vi "e.gate HighSpeedPort Decode TimeStamp.vi"(0 "Data in (binary)":u8[](array[numeric]), 1 "Time Format String":string, 2 "dActTimeDataType":i32, 3 "StartTimeToDayFactor":dbl, 4 "dActTimeToSecondFactor":dbl, 5 "StartTime":dbl, 7 "error in (no error)":errorcluster, 15 "Array":dbl[](array[numeric])) -> (20 "OLE time":dbl, 21 "date time array (double)":dbl[](array[numeric]), 22 "date time cluster":T1 caption="date time rec", 27 "error out":cluster{"status":bool, i32, "source":string})   [LabVIEW 2016]
doc: "This VI is used to decode the timestamp of a buffer frame depending on calculated time information's from the controller and a Time Format String which defines the time/date information's to be inserted in the output array."
uses:
  <vilib>/Utility/miscctls.llb/LVDateTimeRec.ctl
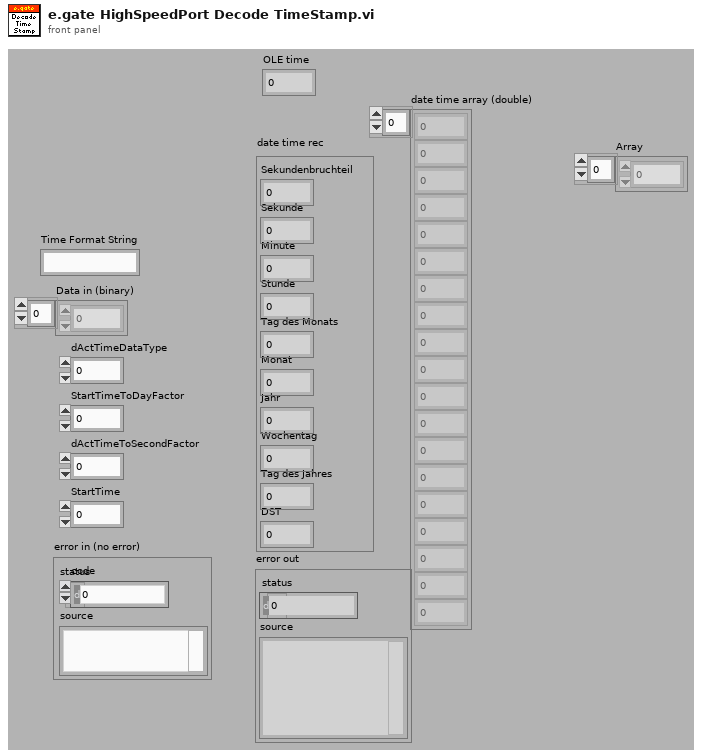
[diagram p1: front panel]
types:
  T1 = typedef "LVDateTimeRec.ctl" = cluster{"fractional second":dbl, "second":i32, "minute":i32, "hour":i32, "day of month":i32, "month":i32, "year":i32, "day of week":i32, "day of year":i32, "DST":i32}
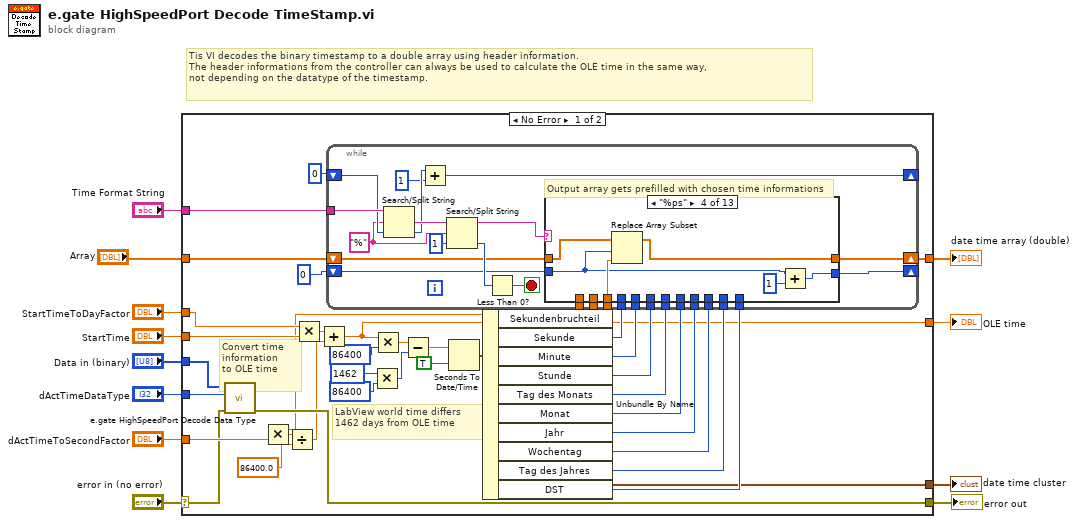
[diagram p0: block diagram]
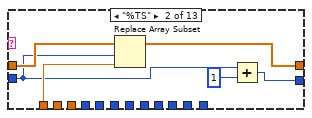
[diagram p3: hidden frame]
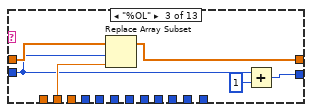
[diagram p4: hidden frame]
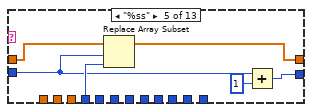
[diagram p5: hidden frame]
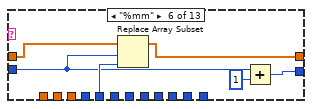
[diagram p6: hidden frame]
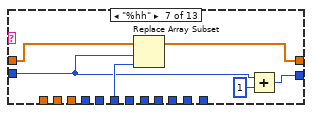
[diagram p7: hidden frame]
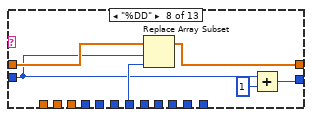
[diagram p8: hidden frame]
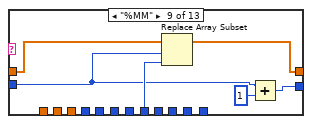
[diagram p9: hidden frame]
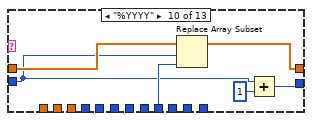
[diagram p10: hidden frame]
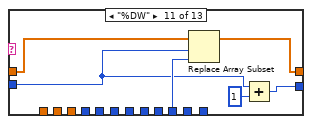
[diagram p11: hidden frame]
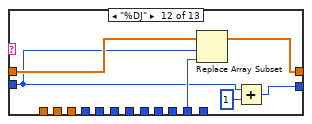
[diagram p12: hidden frame]
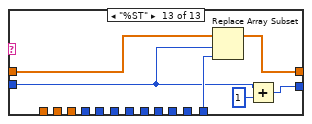
[diagram p13: hidden frame]
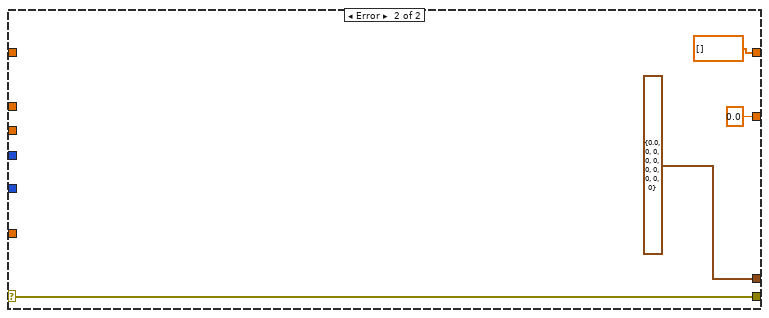
[diagram p14: hidden frame]
diagram:
  # "Tis VI decodes the binary timestamp to a double array using header information.\nThe header informations from the controller can always be used to calculate the OLE time in the same way,\nnot depending on the datatype of the timestamp."
  n1 = case shown="No Error" "error in (no error)" {
    selector: "error in (no error)" -> [w16 w153]
    tunnel: [w48 w153] -> w12
    tunnel: "dActTimeDataType" -> [w15 _]
    tunnel: "StartTime" -> [w47 _]
    tunnel: "dActTimeToSecondFactor" -> [w46 _]
    tunnel: "Data in (binary)" -> [w17 _]
    tunnel: "StartTimeToDayFactor" -> [w34 _]
    tunnel: "Time Format String" -> [w19 _]
    tunnel: [w23 0.0] -> w5
    tunnel: [w22 dbl[] [] ("Angehängtes Array")] -> w3
    tunnel: [w21 T1 {"fractional second"=0.0, "second"=0, "minute"=0, "hour"=0, "day of month"=0, "month"=0, "year"=0, "day of week"=0, "day of year"=0, "DST"=0} ("date time rec")] -> w2
    tunnel: "Array" -> [w14 _]
    frame No Error {
      # "Convert time \ninformation\nto OLE time"
      # "LabView world time differs\n1462 days from OLE time"
      n2 = call "e.gate HighSpeedPort Decode Data Type.vi"("error in (no errro)"=w16, "DataTypeIndex"=w15, "data in (binary)"=w17) -> ("error out"=w48:errorcluster, "value (double)"=w20:dbl)  [unwired: 1 in, 6 out]
      n3 = Multiply(x=w20, y=w46) -> (x*y=w36:dbl)
      n4 = Divide(x=w36, y=86400.0) -> (x/y=w35:dbl)
      n5 = Multiply(x=w34, y=w47) -> (x*y=w38:dbl)
      n6 = Add ("Addieren")(x=w38, y=w35) -> (x+y=w23:dbl)
      n7 = Multiply(x=1462 ("y"), y=86400) -> (x*y=w41:i32)
      n8 = Multiply(x=w23, y=86400) -> (x*y=w43:dbl)
      n9 = Subtract(x=w43, y=w41) -> (x-y=w44:dbl)
      n10 = Seconds To Date/Time(time stamp (now)=w44, to UTC (F)=TRUE ("in Weltzeit (F)")) -> (date time rec=w21:T1)
      n11 = Unbundle By Name(w21) -> ("Sekundenbruchteil"=w33:dbl, "Sekunde"=w32:i32, "Minute"=w31:i32, "Stunde"=w30:i32, "Tag des Monats"=w29:i32, "Monat"=w28:i32, "Jahr"=w27:i32, "Wochentag"=w26:i32, "Tag des Jahres"=w25:i32, "DST"=w24:i32)
      n12 = while {
        shift-right: [w75] -> w22
        shift-left: w14 -> [w51]
        tunnel: w33 -> [w74]
        tunnel: w32 -> [w73]
        tunnel: w31 -> [w72]
        tunnel: w30 -> [w71]
        tunnel: w29 -> [w70]
        tunnel: w28 -> [w69]
        tunnel: w27 -> [w68]
        tunnel: w26 -> [w67]
        tunnel: w25 -> [w66]
        tunnel: w24 -> [w65]
        tunnel: w23 -> [w64]
        tunnel: w20 -> [w63]
        tunnel: w19 -> [w62]
        shift-right: [w54] -> _
        shift-left: 0 ("offset of match") -> [w61]
        shift-right: [w49] -> _
        shift-left: 0 ("offset of match") -> [w50]
        stop <- w56 stop-if-true
        w58 = "%" ("Nach String/Zeichen suchen (-)")
        # "Output array gets prefilled with chosen time informations"
        n13 = Search/Split String(string=w62, search string/char (-)=w58, offset (0)=w61) -> (match + rest of string=w60:string, offset of match=w53:i32)  [unwired: 1 out]
        n14 = Add ("Addieren")(x=w53, y=1) -> (x+y=w54:i32)
        n15 = Search/Split String(string=w60, search string/char (-)=w58, offset (0)=1 ("Offset (0)")) -> (substring before match=w57:string, offset of match=w55:i32)  [unwired: 1 out]
        n16 = Less Than 0?(x=w55) -> (x < 0?=w56:bool)
        n17 = case shown="\"%ps\"" w57 {
          tunnel: w51 -> [w77 w83 w86 w94 w98 w107 w112 w118 w124 w130 w136 w142 w148]
          tunnel: [w77 w81 w84 w93 w97 w102 w111 w117 w120 w129 w135 w141 w147] -> w75
          tunnel: w74 -> [_ _ _ w95 _ _ _ _ _ _ _ _ _]
          tunnel: w73 -> [_ _ _ _ w99 _ _ _ _ _ _ _ _]
          tunnel: w72 -> [_ _ _ _ _ w106 _ _ _ _ _ _ _]
          tunnel: w71 -> [_ _ _ _ _ _ w113 _ _ _ _ _ _]
          tunnel: w70 -> [_ _ _ _ _ _ _ w119 _ _ _ _ _]
          tunnel: w69 -> [_ _ _ _ _ _ _ _ w125 _ _ _ _]
          tunnel: w68 -> [_ _ _ _ _ _ _ _ _ w131 _ _ _]
          tunnel: w67 -> [_ _ _ _ _ _ _ _ _ _ w137 _ _]
          tunnel: w66 -> [_ _ _ _ _ _ _ _ _ _ _ w143 _]
          tunnel: w65 -> [_ _ _ _ _ _ _ _ _ _ _ _ w149]
          tunnel: w64 -> [_ _ w87 _ _ _ _ _ _ _ _ _ _]
          tunnel: w63 -> [_ w82 _ _ _ _ _ _ _ _ _ _ _]
          tunnel: w50 -> [w76 w80 w85 w90 w96 w103 w109 w115 w122 w127 w133 w139 w145]
          tunnel: [w76 w79 w88 w91 w100 w104 w108 w114 w121 w126 w132 w138 w144] -> w49
          frame "", Default {
          }
          frame "%TS" {
            n18 = Replace Array Subset(array=w83, new element=w82, index=w80) -> (w81:dbl[])
            n19 = Add(x=w80, y=1) -> (x+y=w79:i32)
          }
          frame "%OL" {
            n20 = Replace Array Subset(array=w86, new element=w87, index=w85) -> (w84:dbl[])
            n21 = Add(x=w85, y=1) -> (x+y=w88:i32)
          }
          frame "%ps" {
            n22 = Replace Array Subset(array=w94, new element=w95, index=w90) -> (w93:dbl[])
            n23 = Add(x=w90, y=1) -> (x+y=w91:i32)
          }
          frame "%ss" {
            n24 = Replace Array Subset(array=w98, new element=w99, index=w96) -> (w97:dbl[])
            n25 = Add(x=w96, y=1) -> (x+y=w100:i32)
          }
          frame "%mm" {
            n26 = Replace Array Subset(array=w107, new element=w106, index=w103) -> (w102:dbl[])
            n27 = Add(x=w103, y=1) -> (x+y=w104:i32)
          }
          frame "%hh" {
            n28 = Replace Array Subset(array=w112, new element=w113, index=w109) -> (w111:dbl[])
            n29 = Add(x=w109, y=1) -> (x+y=w108:i32)
          }
          frame "%DD" {
            n30 = Replace Array Subset(array=w118, new element=w119, index=w115) -> (w117:dbl[])
            n31 = Add(x=w115, y=1) -> (x+y=w114:i32)
          }
          frame "%MM" {
            n32 = Replace Array Subset(array=w124, new element=w125, index=w122) -> (w120:dbl[])
            n33 = Add(x=w122, y=1) -> (x+y=w121:i32)
          }
          frame "%YYYY" {
            n34 = Replace Array Subset(array=w130, new element=w131, index=w127) -> (w129:dbl[])
            n35 = Add(x=w127, y=1) -> (x+y=w126:i32)
          }
          frame "%DW" {
            n36 = Replace Array Subset(array=w136, new element=w137, index=w133) -> (w135:dbl[])
            n37 = Add(x=w133, y=1) -> (x+y=w132:i32)
          }
          frame "%DJ" {
            n38 = Replace Array Subset(array=w142, new element=w143, index=w139) -> (w141:dbl[])
            n39 = Add(x=w139, y=1) -> (x+y=w138:i32)
          }
          frame "%ST" {
            n40 = Replace Array Subset(array=w148, new element=w149, index=w145) -> (w147:dbl[])
            n41 = Add(x=w145, y=1) -> (x+y=w144:i32)
          }
        }
      }
    }
    frame Error {
    }
  }
  "OLE time" <- w5
  "error out" <- w12
  "date time array (double)" <- w3
  "date time cluster" <- w2
